vi "load login credentials.vi"(8 "error in":errorcluster, 10 "device model":enum16{"cRIO-9068"}(ring)) -> (0 "error out":errorcluster, 3 "login credentials":T1)   [LabVIEW 2014]
uses:
  <vilib>/Utility/config.llb/NI_LVConfig.lvlib
  <vilib>/Utility/config.llb/Read Key (String).vi
  login credentials.ctl
  tests.lvlib
panel:
  out "login credentials 2":T1[](array[typedef])
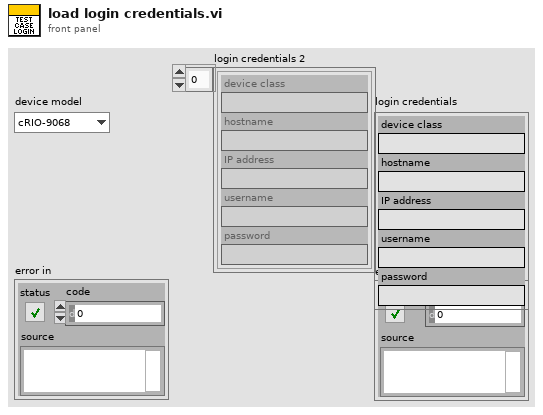
[diagram p1: front panel]
types:
  T1 = typedef "tests.lvlib/login credentials.ctl" = cluster{"device class":string, "hostname":string, "IP address":string, "username":string, "password":string}
  T2 = typedef "SMI.lvlib/Device.lvclass/login credentials.ctl" = cluster{"device class":string, "hostname":string, "IP address":string, "username":string, "password":string}
  T3 = typedef "NI_LVConfig.lvlib/Config Data RefNum.ctl" = refnum<k1>
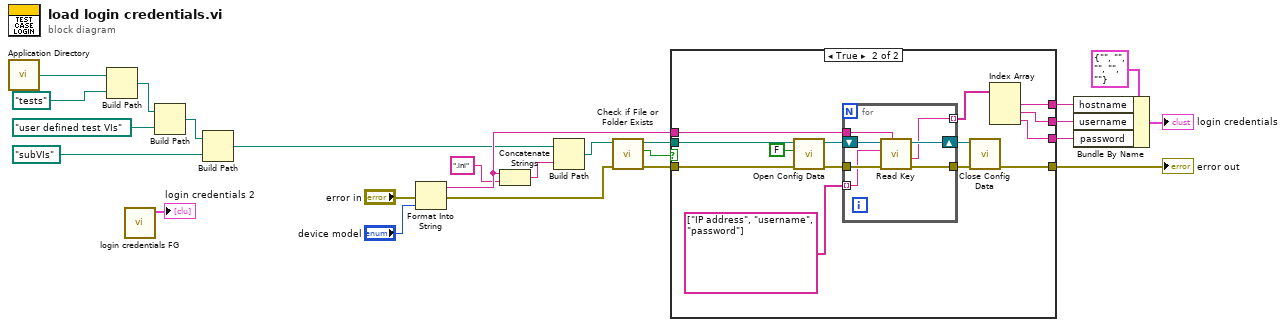
[diagram p0: block diagram]
diagram:
  n1 = call <vilib>:"Application Directory.vi"() -> ("Application Directory"=w12:path)
  n2 = Build Path(base path=w12, name or relative path=path "tests") -> (appended path=w10:path)
  n3 = call "login credentials FG.vi"() -> ("login credentials"=→"login credentials 2":T2[])  [unwired: 10 in, 1 out]
  n4 = Build Path(base path=w10, name or relative path=path "user defined test VIs") -> (appended path=w7:path)
  n5 = Build Path(base path=w7, name or relative path=path "subVIs") -> (appended path=w13:path)
  n6 = Format Into String(error in="error in", "device model") -> (resulting string=w23:string, error out=w20:errorcluster)  [unwired: 2 in]
  n7 = Concatenate Strings(w23, ".ini" ("string")) -> (w14:string)
  n8 = Build Path(base path=w13, name or relative path=w14) -> (appended path=w22:path)
  n9 = call <vilib>:"Check if File or Folder Exists.vi"("error in (no error)"=w20, "path"=w22) -> ("error out"=w19:errorcluster, "file or folder exists?"=w18:bool, "dup path"=w21:path)  [unwired: 7 in]
  n10 = case shown="True" w18 {
    tunnel: [w25 w35] -> w24
    tunnel: [_ w31] -> w5
    tunnel: [_ w30] -> w4
    tunnel: [_ w29] -> w3
    tunnel: w23 -> [_ w28]
    tunnel: w21 -> [_ w27]
    tunnel: w19 -> [w25 w26]
    frame False {
    }
    frame True {
      n11 = call <vilib>:"Open Config Data.vi"("error in (no error)"=w26, "create file if necessary (T)"=FALSE, "configuration file path"=w27) -> ("error out"=w37:errorcluster, "refnum"=w38:T3)  [unwired: 6 in, 1 out]
      n12 = for {
        tunnel: w37 -> [w45]
        tunnel: w28 -> [w44]
        tunnel: string[] ["IP address", "username", "password"] -> [w43] mode=indexing
        shift-right: [w42] -> w33
        shift-left: w38 -> [w46]
        tunnel: [w41] -> w34
        tunnel: [w40] -> w32 mode=indexing
        n13 = call-poly <vilib>:"Read Key.vi"("section"=w44, "error in (no error)"=w45, "key"=w43, "refnum"=w46) -> ("error out"=w41:errorcluster, "value"=w40:string, "refnum out"=w42:T3)  [unwired: 4 in, 1 out]
      }
      n14 = call <vilib>:"Close Config Data.vi"("error in (no error)"=w34, "refnum"=w33) -> ("error out"=w35:errorcluster)  [unwired: 8 in, 1 out]
      n15 = Index Array(array=w32) -> (element #1=w31:string, element #2=w30:string, element #3=w29:string)  [unwired: 3 in]
    }
  }
  "error out" <- w24
  n16 = Bundle By Name(cluster=T1 {"device class"="", "hostname"="", "IP address"="", "username"="", "password"=""} ("login credentials"), "hostname"=w5, "username"=w4, "password"=w3) -> (→"login credentials":T1)
